vi "Sweep Voltage.vi"() -> ()   [LabVIEW 2009, in "LCD Retarder.lvclass"]
uses:
  LCD Retarder.lvclass
  DAQ/DAQmx Analog.lvclass
  Utility Classes/Readable/Readable.lvclass
  <vilib>/Analysis/NI_AALBase.lvlib
panel:
  out "Smoothed Graph":cluster{"Y":dbl[], "Y":dbl[]}[](graph)
  out "Run #":dbl
  in  "Averages":dbl
  out "Current Retardance":dbl[unit]
  out "?":dbl
  out "Minimum":dbl
  in  "Analog DAQ Ch#":i32
  in  "Ending Voltage":dbl
  in  "Starting Voltage":dbl
  out "LCD curve":cluster{"Y":dbl[], "Y":dbl[]}[](graph)
  # "at LCD Voltage"
  # "V"
  # "Volts"
  # "Volts"
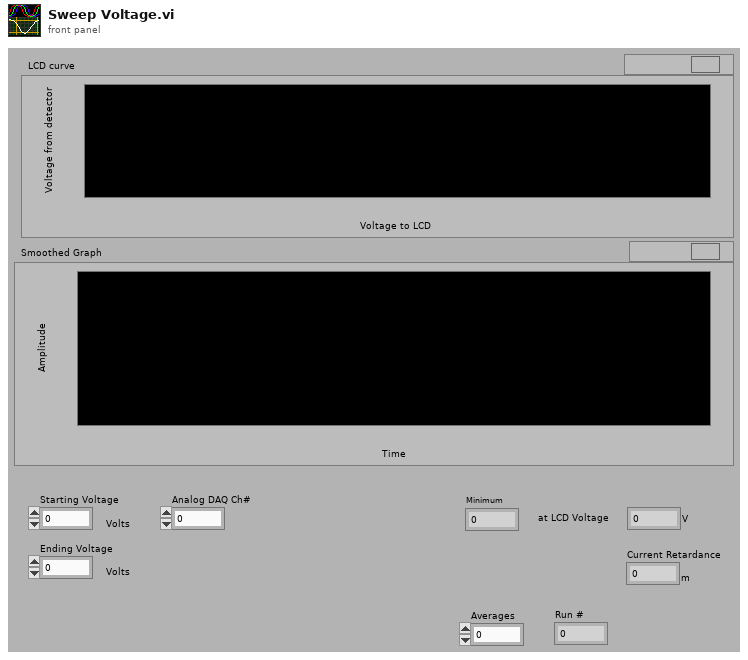
[diagram p1: front panel]
types:
  T1 = typedef "Readable.lvclass/X array.ctl" = T2[]
  T2 = typedef "Readable.lvclass/X.ctl" = dbl
  T3 = cluster{"Channel Names[0]":string, "Channel Names[1]":string, "Channel Names[2]":string, "Channel Names[3]":string, "Channel Names[4]":string, "Channel Names[5]":string, "Channel Names[6]":string, "Channel Names[7]":string, "Channel Names[8]":string}
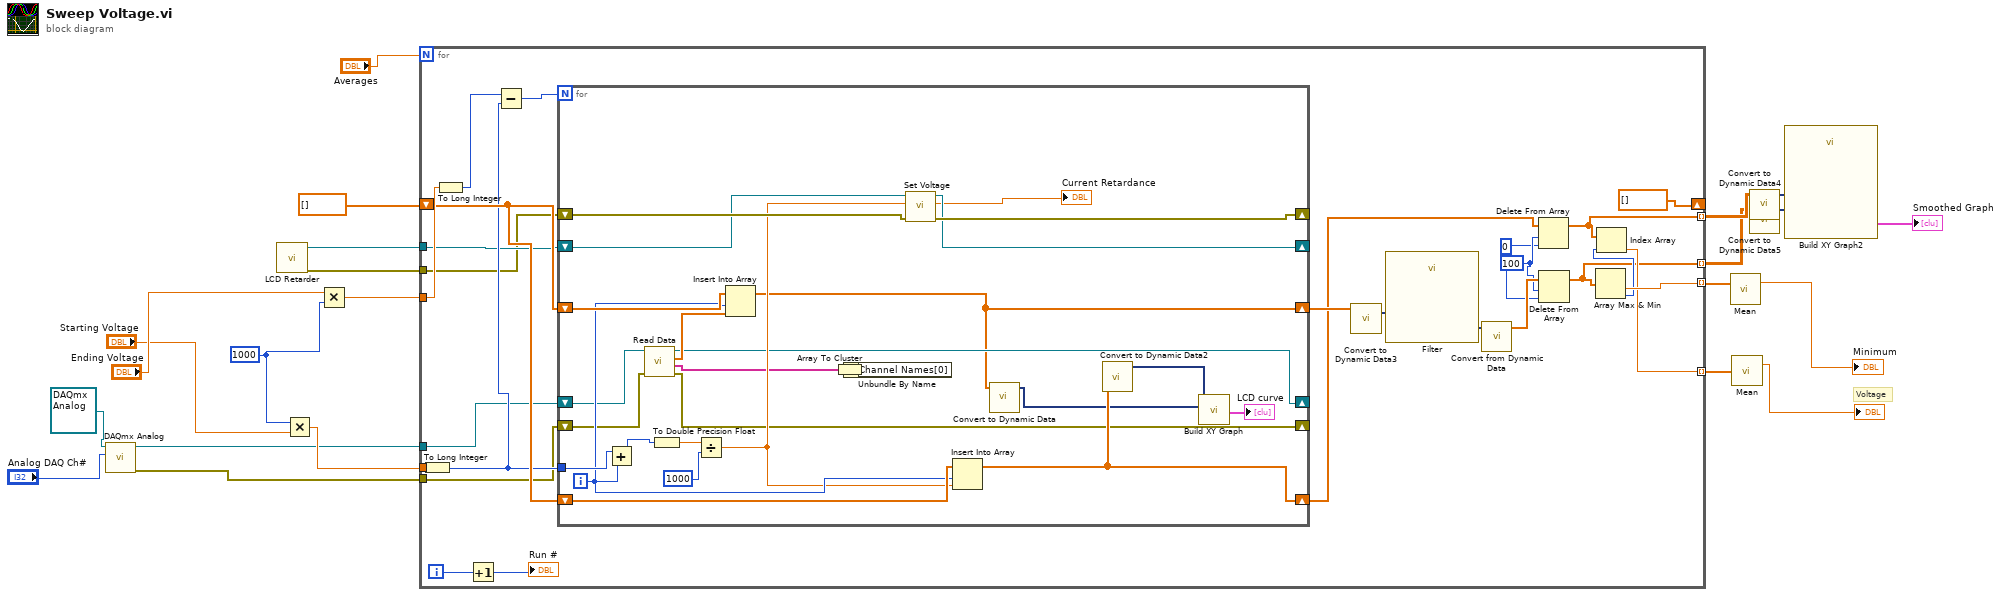
[diagram p0: block diagram]
diagram:
  w22 = 1000
  # "Voltage"
  n1 = call "DAQmx Analog.vi"("Analog input #"="Analog DAQ Ch#", "DAQmx Analog in"=refnum<class "DAQmx Analog.lvclass"> refnum ("DAQmx Analog.lvclass")) -> ("error out"=w12:errorcluster, "DAQmx Analog out"=w13:refnum<class "DAQmx Analog.lvclass">)  [unwired: 8 in]
  n2 = call "LCD Retarder.vi"() -> ("errorOUT"=w14:errorcluster, "LCD out"=w15:refnum<class "LCD Retarder.lvclass">)  [unwired: 10 in]
  n3 = Multiply(x=w22, y="Starting Voltage") -> (x*y=w21:dbl)
  n4 = Multiply(x="Ending Voltage", y=w22) -> (x*y=w20:dbl)
  n5 = for {
    N: "Averages" -> [_]
    tunnel: w21 -> [w47]
    tunnel: w20 -> [w45]
    tunnel: w15 -> [w41]
    tunnel: w14 -> [w40]
    tunnel: w13 -> [w39]
    tunnel: w12 -> [w38]
    shift-right: [dbl[] []] -> _
    shift-left: dbl[] [] -> [w44]
    tunnel: [w37] -> w9 mode=indexing
    tunnel: [w25] -> w3 mode=indexing
    tunnel: [w24] -> w2 mode=indexing
    tunnel: [w23] -> w1 mode=indexing
    i -> [w35]
    w28 = 100
    w27 = 0
    n6 = To Long Integer(number=w47) -> (32bit integer=w42:i32)
    n7 = To Long Integer(number=w45) -> (32bit integer=w46:i32)
    n8 = Increment(x=w35) -> (x+1=→"Run #":i32)
    n9 = Subtract(x=w46, y=w42) -> (x-y=w43:i32)
    n10 = for {
      N: w43 -> [_]
      shift-right: [w51] -> _
      shift-left: w39 -> [w60]
      shift-right: [w57] -> _
      shift-left: w40 -> [w63]
      shift-right: [w56] -> _
      shift-left: w41 -> [w61]
      shift-right: [w50] -> _
      shift-left: w38 -> [w59]
      tunnel: w42 -> [w68]
      shift-right: [w48] -> w33
      shift-left: w44 -> [w67]
      shift-right: [w64] -> w31
      shift-left: w44 -> [w66]
      i -> [w65]
      n11 = Add(x=w68, y=w65) -> (x+y=w69:i32)
      n12 = call "Read Data.vi"("error in (no error)"=w59, "Readable in"=w60) -> ("error out"=w50:errorcluster, "Channel Names"=w58:string[], "X array"=w52:T1, "Readable out"=w51:refnum<class "DAQmx Analog.lvclass">)  [unwired: 3 in, 3 out]
      n13 = To Double Precision Float(number=w69) -> (double precision float=w71:dbl)
      n14 = Divide(x=w71, y=1000) -> (x/y=w62:dbl)
      n15 = Insert Into Array(array=w67, index=w65, new element=w52) -> (w48:dbl[])
      n16 = Array To Cluster(array=w58) -> (cluster=w72:T3)
      n17 = Unbundle By Name(w72) -> ()  [unwired: 1 out]
      n18 = call "Set Voltage.vi"("errorIN"=w63, "Voltage in"=w62, "LCD in"=w61) -> ("errorOUT"=w57:errorcluster, "Retardance out"=→"Current Retardance":dbl[unit], "LCD out"=w56:refnum<class "LCD Retarder.lvclass">)  [unwired: 6 in]
      n19 = Insert Into Array(array=w66, index=w65, new element=w62) -> (w64:dbl[])
      n20 = call "Convert to Dynamic Data"("Array"=w48) -> ("Dynamic Data Type"=w54:dynamicdata)  [unwired: 3 in]
      n21 = call "Convert to Dynamic Data2"("Array"=w64) -> ("Dynamic Data Type"=w55:dynamicdata)  [unwired: 3 in]
      n22 = call "Build XY Graph"("Y Input"=w54, "X Input"=w55) -> ("XY Graph"=→"LCD curve":cluster{"Y":dbl[], "Y":dbl[]}[])  [unwired: 8 in, 1 out]
    }
    n23 = call "Convert to Dynamic Data3"("Array"=w33) -> ("Dynamic Data Type"=w32:dynamicdata)  [unwired: 3 in]
    n24 = call "Filter"("Signal"=w32) -> ("Filtered Signal"=w30:dynamicdata)  [unwired: 9 in, 1 out]
    n25 = call "Convert from Dynamic Data"("Dynamic Data Type"=w30) -> ("Array"=w29:dbl[])  [unwired: 3 in]
    n26 = Delete From Array(array=w31, length=w28, index=w27) -> (array with subset deleted=w24:dbl[])  [unwired: 1 out]
    n27 = Delete From Array(array=w29, length=w28, index=w27) -> (array with subset deleted=w23:dbl[])  [unwired: 1 out]
    n28 = Array Max & Min(array=w23) -> (min value=w37:dbl, min index (indices)=w26:i32)  [unwired: 2 out]
    n29 = Index Array(array=w24, index=w26) -> (element=w25:dbl)
  }
  n30 = call <vilib>:"Mean.vi"("X"=w9) -> ("mean"=→"Minimum":dbl)  [unwired: 1 out]
  n31 = call <vilib>:"Mean.vi"("X"=w3) -> ("mean"=→"?":dbl)  [unwired: 1 out]
  n32 = call "Convert to Dynamic Data4"("2D Array"=w2) -> ("Dynamic Data Type"=w5:dynamicdata)  [unwired: 3 in]
  n33 = call "Convert to Dynamic Data5"("2D Array"=w1) -> ("Dynamic Data Type"=w4:dynamicdata)  [unwired: 3 in]
  n34 = call "Build XY Graph2"("Y Input"=w4, "X Input"=w5) -> ("XY Graph"=→"Smoothed Graph":cluster{"Y":dbl[], "Y":dbl[]}[])  [unwired: 8 in, 1 out]
